vi "send_command.vi"(2 "错误输入":errorcluster caption="错误输入（无错误）", 3 "command in":u8[](array[numeric]), 4 "com in":refnum<visa-resource-name>) -> (0 "错误输出":errorcluster, 1 "com out":refnum<visa-resource-name>)   [LabVIEW 2018]
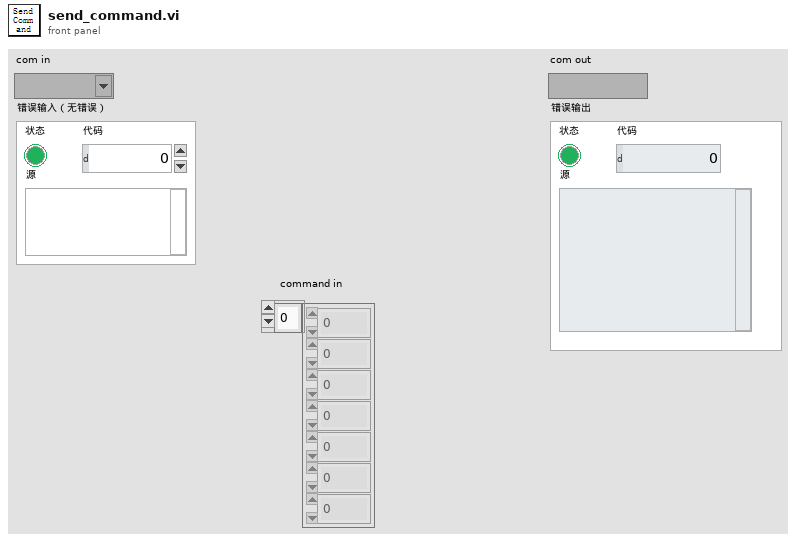
[diagram p1: front panel]
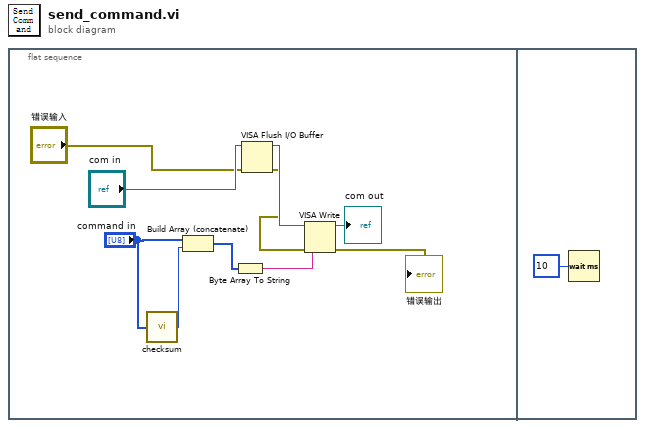
[diagram p0: block diagram]
diagram:
  n1 = flat-sequence {
    frame #0 {
      n2 = call "checksum.vi"("data"="command in") -> ("checksum"=w9:u8)
      n3 = Build Array (concatenate)("command in", w9) -> (w8:u8[])
      n4 = Byte Array To String(unsigned byte array=w8) -> (string=w7:string)
      n5 = VISA Flush I/O Buffer(VISA resource name="com in", error in (no error)="错误输入") -> (VISA resource name out=w2:refnum<visa-resource-name>, error out=w1:errorcluster)  [unwired: 1 in]
      n6 = VISA Write(VISA resource name=w2, write buffer=w7, error in (no error)=w1) -> (VISA resource name out=→"com out":refnum<visa-resource-name>, error out=→"错误输出":errorcluster)  [unwired: 1 out]
    }
    frame #1 {
      n7 = Wait (ms)(milliseconds to wait=u32 10 ("等待时间（毫秒）")) -> ()  [unwired: 1 out]
    }
  }
